vi "Write I32 Array.vi"(8 "error in (no error)":errorcluster, 10 "I32 Array":i32[][](array[numeric]), 11 "Scaled I32 Array Result in":refnum<class "Scaled I32 Array Result.lvclass">) -> (0 "error out":errorcluster, 3 "Scaled I32 Array Result out":refnum<class "Scaled I32 Array Result.lvclass">)   [LabVIEW 2015, in "Scaled I32 Array Result.lvclass"]
uses:
  Scaled I32 Array Result.lvclass
  Scaled I32 Array Result.lvclass/Scaled I32 Array Result.ctl
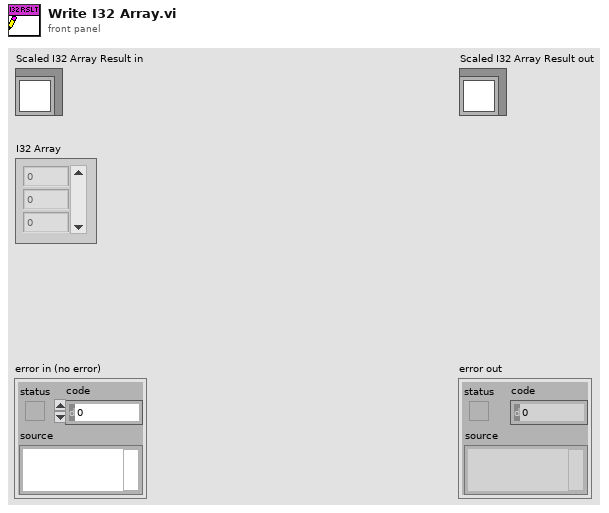
[diagram p1: front panel]
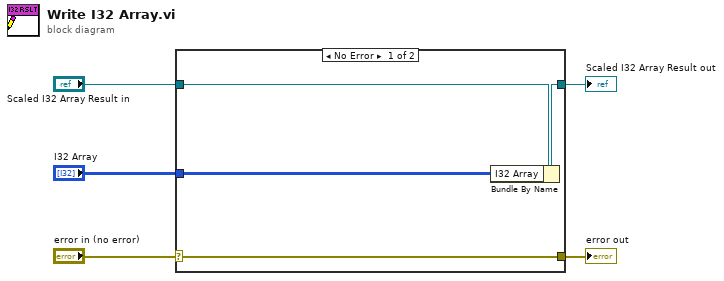
[diagram p0: block diagram]
diagram:
  n1 = case shown="No Error" "error in (no error)" {
    selector: "error in (no error)" -> [w9 w10]
    tunnel: [w9 w10] -> w4
    tunnel: [w7 w11] -> w2
    tunnel: "Scaled I32 Array Result in" -> [w8 w11]
    tunnel: "I32 Array" -> [w6 _]
    frame No Error {
      n2 = Bundle By Name(cluster=w8, "I32 Array"=w6) -> (w7:refnum<class "Scaled I32 Array Result.lvclass">)
    }
    frame Error {
    }
  }
  "error out" <- w4
  "Scaled I32 Array Result out" <- w2
